vi "Autonomous Independent.vi"() -> ()   [LabVIEW 2019]
doc: "This VI is called when autonomous begins, and will automatically be terminated when autonomous ends. You can carry out timed or sensor driven robot movement independently without needing to return to the caller."
uses:
  <vilib>/Rock Robotics/Network Tables/NT Read String.vi
  Refnums.vi
  <vilib>/Rock Robotics/WPI/ThirdParty/Phoenix-LabVIEW/Motor Controller/Get/CTRE_Phoenix_MotorController_GetQuadratureData.vi
  <vilib>/addons/control/pid/pid.llb/PID (DBL).vi
  <vilib>/Rock Robotics/WPI/RobotDrive/WPI_RobotDriveArcadeDrive_Standard(NoSaturation).vi
  <vilib>/addons/control/pid/NI_PID_pid.lvlib
panel:
  in  "Autonomous Step":T1(array[cluster]) {"Speed" min=0.0 max=1.0 step=0.01}
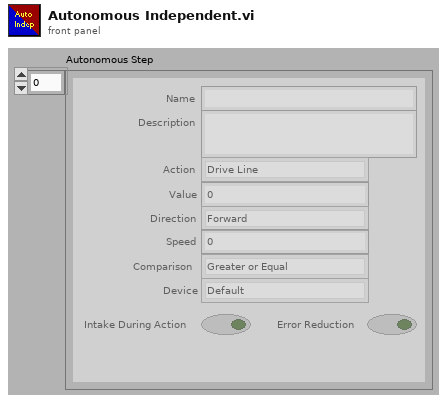
[diagram p1: front panel]
types:
  T1 = cluster{"Name":string, "Description":string, "Action":enum16{"Drive Line", "Drive Turn", "Drive Stop", "Drive Wait", "Shoot", "Motion Profile", ""}, "Value":dbl, "Direction":enum16{"Forward", "Reverse", "Left", "Right"}, "Speed":dbl, "Comparison":enum16{"Greater or Equal", "Less or Equal", "No compare (fixed)"}, "Device":enum16{"Default", "Gyro", "Laser", "Lidar", "Lime Light", "Encoder"}, "Intake During Action":bool, "Error Reduction":bool}[]
  T2 = typedef "WPI_RobotDriveDevRef.ctl" = cluster{"DevStatus":errorcluster, "Motors[]":T3[], "Square Inputs":bool, "Max Output":dbl}
  T3 = typedef "WPI_MotorControlDeviceRef.ctl" = cluster{"DeviceStatus":errorcluster, "Type":T4, "PWM":cluster{"PWM Channel":T5, "DeadBand":T6}, "CAN":cluster{"Device Number":u8, "SetOutput VI Ref":variant, "GetOutput VI Ref":variant, "Enable VI Ref":variant, "Disable VI Ref":variant, "Data":variant}, "Invert":bool, "DIO PWM":cluster{"PWM \"Enable\" Channel":T5, "DIOChannel":T7, "PWM Rate":dbl}}
  T4 = typedef "WPI_MotorControlType.ctl" = enum16{"PWM", "CAN", "DIO PWM"}
  T5 = typedef "FPGA_DIOPWMChannel.ctl" = enum8{"PWM 0", "PWM 1", "PWM 2", "PWM 3", "PWM 4", "PWM 5", "PWM 6", "PWM 7", "PWM 8", "PWM 9", "PWM MXP 0", "PWM MXP 1", "PWM MXP 2", "PWM MXP 3", "PWM MXP 4", "PWM MXP 5", "PWM MXP 6", "PWM MXP 7", "PWM MXP 8", "PWM MXP 9", "Invalid"}
  T6 = typedef "WPI_PWMDeadband.ctl" = cluster{"Name":string, "maxPositivePwm":i32, "minPositivePwm":i32, "centerPwm":i32, "maxNegativePwm":i32, "minNegativePwm":i32, "angularRange":u16}
  T7 = typedef "FPGA_DIOChannel.ctl" = enum8{"DIO 0", "DIO 1", "DIO 2", "DIO 3", "DIO 4", "DIO 5", "DIO 6", "DIO 7", "DIO 8", "DIO 9", "DIO MXP 0", "DIO MXP 1", "DIO MXP 2", "DIO MXP 3", "DIO MXP 4", "DIO MXP 5", "DIO MXP 6", "DIO MXP 7", "DIO MXP 8", "DIO MXP 9", "DIO MXP 10", "DIO MXP 11", "DIO MXP 12", "DIO MXP 13", "DIO MXP 14", "DIO MXP 15", "SPI Port CS1", "SPI Port CS2", "SPI Port CS3", "SPI Port MISO", "SPI Port MOSI", "Invalid"}
  T8 = cluster{"ROBOT_DRIVE":T2, "SHOOTER":T3, "RIGHT_DRIVE":T3, "LEFT_DRIVE":T3, "TURRET":T3, "SHOOTER SLAVE":T3, "INTAKE PIVOT":T3}
  T9 = cluster{"proportional gain (Kc)":dbl, "integral time (Ti, min)":dbl, "derivative time (Td, min)":dbl}
  T10 = enum16{"Drive Line", "Drive Turn", "Drive Stop", "Drive Wait", "Shoot", "Motion Profile", ""}
  T11 = enum16{"Greater or Equal", "Less or Equal", "No compare (fixed)"}
  T12 = enum16{"Default", "Gyro", "Laser", "Lidar", "Lime Light", "Encoder"}
  T13 = cluster{"Yaw":dbl, "Roll":dbl, "Pitch":dbl, "Heading":dbl, "Fused Heading":dbl}
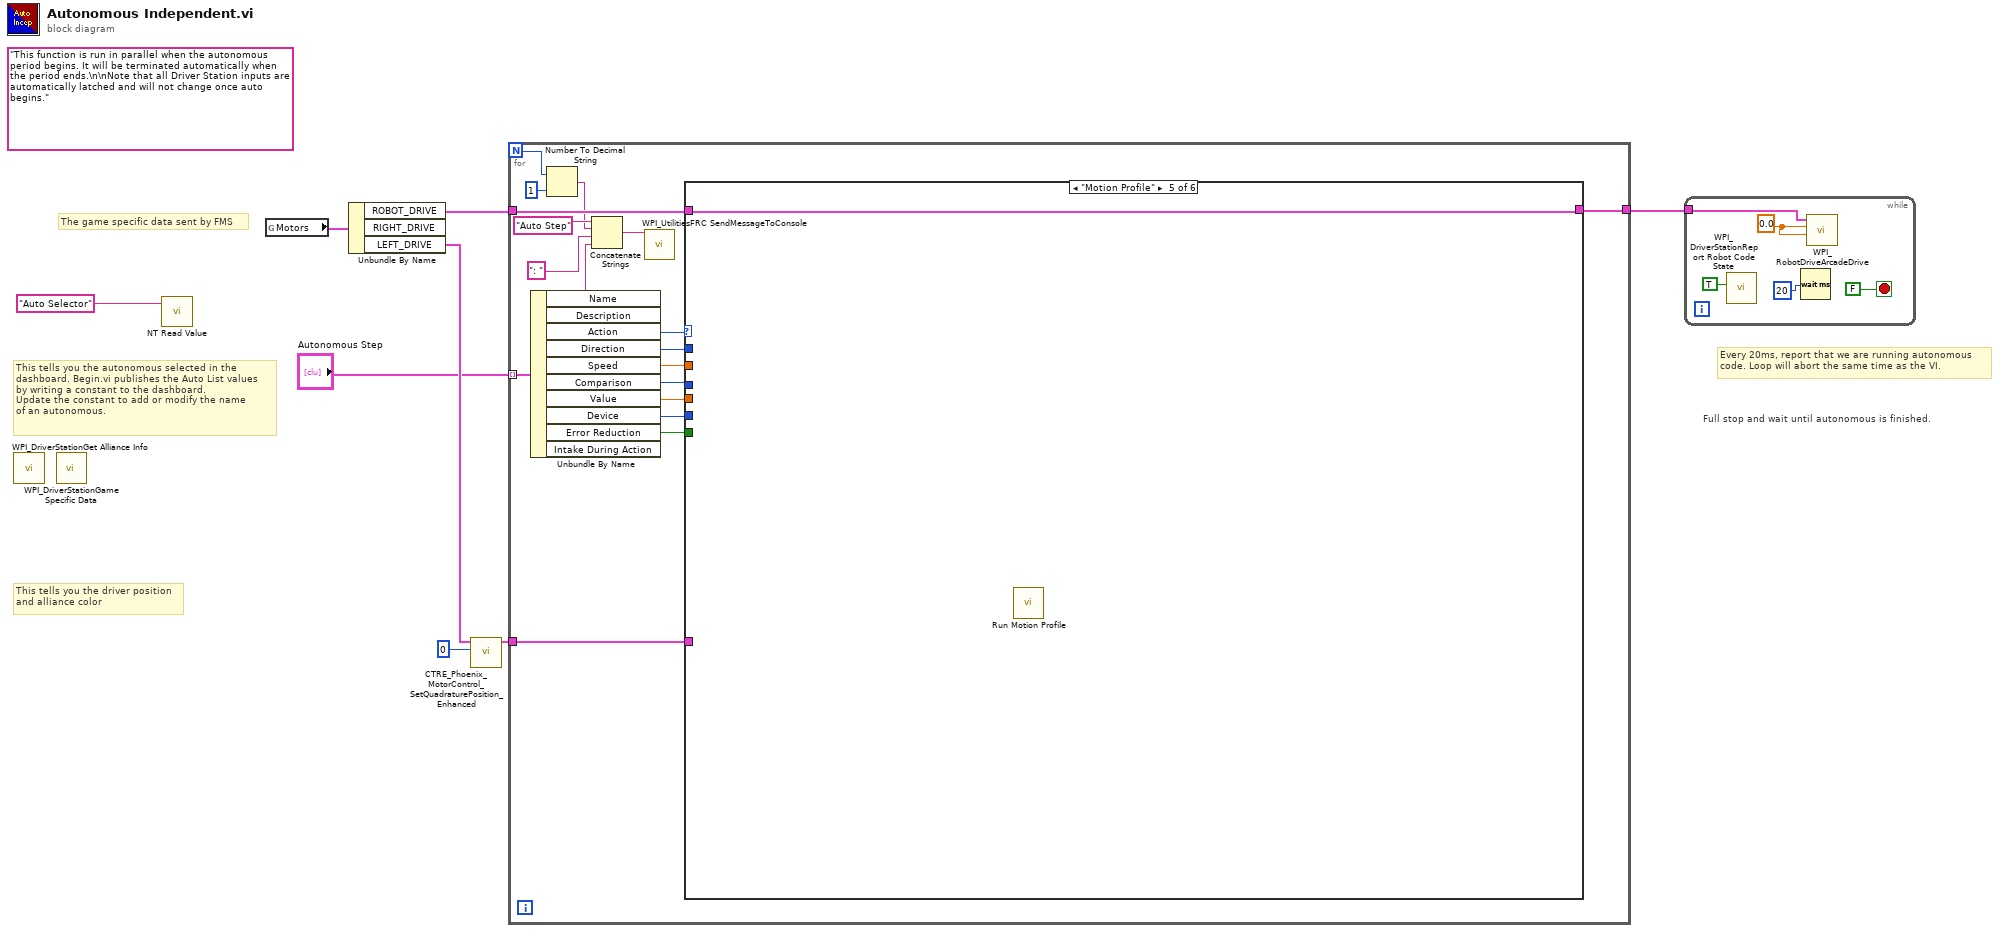
[diagram p0: block diagram]
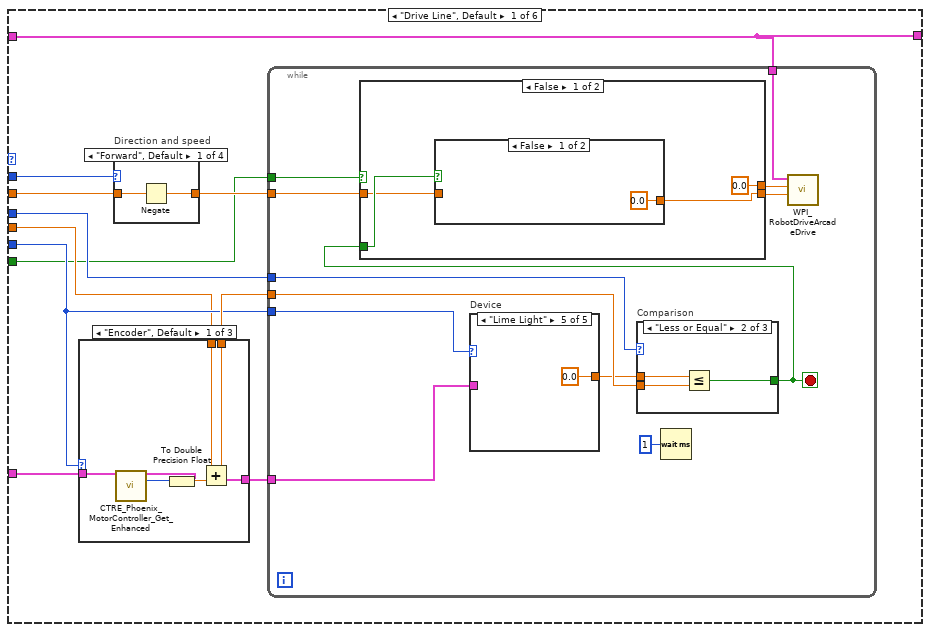
[diagram p2: hidden frame]
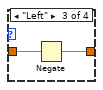
[diagram p6: hidden frame]
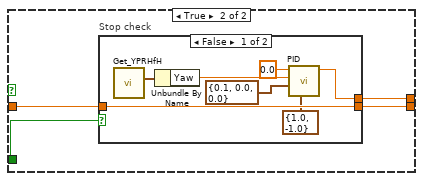
[diagram p9: hidden frame]
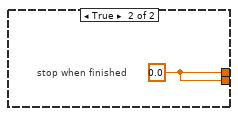
[diagram p10: hidden frame]
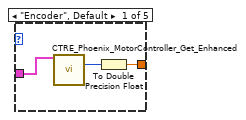
[diagram p11: hidden frame]
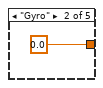
[diagram p12: hidden frame]
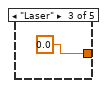
[diagram p13: hidden frame]
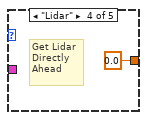
[diagram p14: hidden frame]
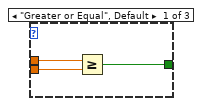
[diagram p15: hidden frame]
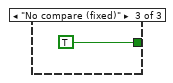
[diagram p16: hidden frame]
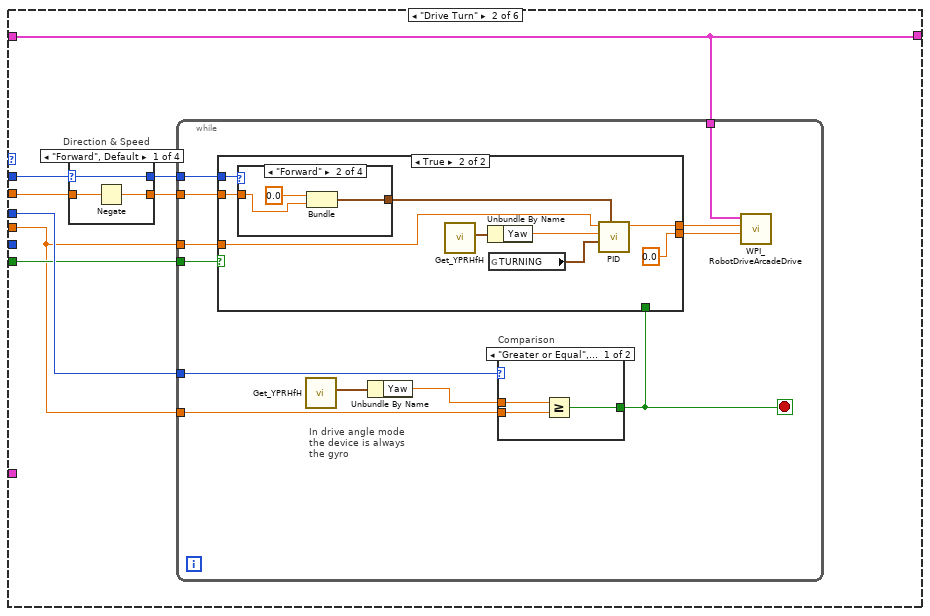
[diagram p17: hidden frame]
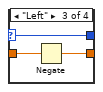
[diagram p19: hidden frame]
diagram:
  (unwired) "This function is run in parallel when the autonomous period begins. It will be terminated automatically when the period ends.\n\nNote that all Driver Station inputs are automatically latched and will not change once auto begins."
  # "Full stop and wait until autonomous is finished."
  # "The game specific data sent by FMS"
  # "This tells you the autonomous selected in the \ndashboard. Begin.vi publishes the Auto List values\nby writing a constant to the dashboard.\nUpdate the constant to add or modify the name\nof an autonomous."
  # "Every 20ms, report that we are running autonomous\ncode. Loop will abort the same time as the VI."
  # "This tells you the driver position\nand alliance color"
  n1 = call <vilib>:"WPI_DriverStationGet Alliance Info.vi"() -> ()  [unwired: 12 out]
  n2 = call <vilib>:"WPI_DriverStationGame Specific Data.vi"() -> ()  [unwired: 11 in, 1 out]
  n3 = call-poly <vilib>:"NT Read Value.vi"("Name"="Auto Selector") -> ()  [unwired: 9 in, 2 out]
  n4 = global read "Refnums.vi" "Motors"() -> (w7:T8)
  n5 = Unbundle By Name(w7) -> ("ROBOT_DRIVE"=w4:T2, "LEFT_DRIVE"=w2:T3)  [unwired: 1 out]
  n6 = call <vilib>:"CTRE_Phoenix_MotorControl_SetQuadraturePosition_Enhanced.vi"("New Position"=0, "PhoenixMotorControlDevRef"=w2) -> ("PhoenixMotorControlDevRef"=w5:T3)  [unwired: 8 in, 1 out]
  n7 = for {
    N -> [w11]
    tunnel: "Autonomous Step" -> [w26] mode=indexing
    tunnel: w5 -> [w18]
    tunnel: w4 -> [w17]
    tunnel: [w16] -> w3
    n8 = Unbundle By Name(w26) -> ("Name"=w14:string, "Action"=w25:T10, "Direction"=w24:enum16{"Forward", "Reverse", "Left", "Right"}, "Speed"=w23:dbl, "Comparison"=w19:T11, "Value"=w20:dbl, "Device"=w22:T12, "Error Reduction"=w21:bool)  [unwired: 2 out]
    n9 = Number To Decimal String(number=w11, width (-)=i16 1) -> (decimal integer string=w9:string)
    n10 = Concatenate Strings("Auto Step" ("string"), w9, ": " ("string"), w14) -> (w15:string)
    n11 = call <vilib>:"WPI_UtilitiesFRC SendMessageToConsole.vi"("Message"=w15) -> ()  [unwired: 14 in, 1 out]
    n12 = case shown="\"Motion Profile\"" w25 {
      tunnel: w24 -> [w32 w102 _ _ _ _]
      tunnel: w23 -> [w33 w104 _ _ _ _]
      tunnel: w22 -> [w34 _ _ _ _ _]
      tunnel: w21 -> [w27 w100 _ _ _ _]
      tunnel: w20 -> [w31 w98 _ w164 _ _]
      tunnel: w19 -> [w30 w103 _ _ _ _]
      tunnel: w18 -> [w29 _ _ _ _ _]
      tunnel: w17 -> [w28 w101 w162 w165 w166 w167]
      tunnel: [w28 w101 w162 w165 w166 w167] -> w16
      frame "Drive Line", Default {
        n13 = case shown="\"Encoder\", Default" w34 {
          tunnel: w29 -> [w43 w44 w46]
          tunnel: w31 -> [w40 w45 w47]
          tunnel: [w39 w45 w47] -> w36
          tunnel: [w38 w44 w46] -> w35
          frame "Encoder", Default {
            n14 = call-poly <vilib>:"CTRE_Phoenix_MotorController_Get_Enhanced.vi"("PhoenixMotorControlDevRef"=w43) -> ("PhoenixMotorControlDevRef"=w38:T3, "Quadrature Position"=w41:i32)  [unwired: 11 in, 2 out]
            n15 = To Double Precision Float(number=w41) -> (double precision float=w42:dbl)
            n16 = Add(x=w40, y=w42) -> (x+y=w39:dbl)
          }
          frame "Gyro" {
          }
          frame "Laser" {
          }
        }
        n17 = case "Direction and speed" shown="\"Forward\", Default" w32 {
          tunnel: w33 -> [w48 w50 w51 w53]
          tunnel: [w49 w50 w52 w53] -> w37
          frame "Forward", Default {
            n18 = Negate(x=w48) -> (-x=w49:dbl)
          }
          frame "Reverse" {
          }
          frame "Left" {
            n19 = Negate(x=w51) -> (-x=w52:dbl)
          }
          frame "Right" {
          }
        }
        n20 = while {
          tunnel: w30 -> [w60]
          tunnel: w36 -> [w65]
          tunnel: w37 -> [w64]
          tunnel: w34 -> [w59]
          tunnel: w28 -> [w61]
          tunnel: w35 -> [w57]
          tunnel: w27 -> [w54]
          stop <- w55 stop-if-true
          n21 = case "Device" shown="\"Lime Light\"" w59 {
            tunnel: [w85 0.0 0.0 0.0 0.0] -> w58
            tunnel: w57 -> [w86 _ _ _ _]
            frame "Encoder", Default {
              n22 = call-poly <vilib>:"CTRE_Phoenix_MotorController_Get_Enhanced.vi"("PhoenixMotorControlDevRef"=w86) -> ("Quadrature Position"=w84:i32)  [unwired: 11 in, 3 out]
              n23 = To Double Precision Float(number=w84) -> (double precision float=w85:dbl)
            }
            frame "Gyro" {
            }
            frame "Laser" {
            }
            frame "Lidar" {
              # "Get Lidar \nDirectly \nAhead"
            }
            frame "Lime Light" {
            }
          }
          n24 = case "Comparison" shown="\"Less or Equal\"" w60 {
            tunnel: [w93 w96 TRUE] -> w55
            tunnel: w65 -> [w92 w95 _]
            tunnel: w58 -> [w91 w94 _]
            frame "Greater or Equal", Default {
              n25 = Greater Or Equal?(x=w91, y=w92) -> (x >= y?=w93:bool)
            }
            frame "Less or Equal" {
              n26 = Less Or Equal?(x=w94, y=w95) -> (x <= y?=w96:bool)
            }
            frame "No compare (fixed)" {
            }
          }
          n27 = case shown="False" w54 {
            tunnel: w64 -> [w67 w75]
            tunnel: [0.0 ("X axis value") w74] -> w63
            tunnel: [w66 w73] -> w62
            tunnel: w55 -> [w68 w72]
            frame False {
              n28 = case shown="False" w68 {
                tunnel: w67 -> [_ w71]
                tunnel: [0.0 ("Speed") w71] -> w66
                frame False {
                }
                frame True {
                }
              }
            }
            frame True {
              n29 = case "Stop check" shown="False" w72 {
                tunnel: w75 -> [w82 _]
                tunnel: [w81 w83] -> w74
                tunnel: [w82 w83] -> w73
                frame False {
                  n30 = call <vilib>:"Get_YPRHfH.vi"() -> ("YRPHfH"=w77:T13)  [unwired: 11 in]
                  n31 = Unbundle By Name(w77) -> ("Yaw"=w76:dbl)
                  n32 = call-poly <vilib>:"PID.vi"("output range"=cluster{"output high":dbl, "output low":dbl} {"output high"=1.0, "output low"=-1.0}, "PID gains"=T9 {"proportional gain (Kc)"=0.1, "integral time (Ti, min)"=0.0, "derivative time (Td, min)"=0.0}, "process variable"=w76, "setpoint"=0.0) -> ("output"=w81:dbl)  [unwired: 6 in, 1 out]
                }
                frame True {
                  w83 = 0.0 ("X axis value")
                  # "stop when finished"
                }
              }
            }
          }
          n33 = Wait (ms)(milliseconds to wait=u32 1) -> ()  [unwired: 1 out]
          n34 = call-poly <vilib>:"WPI_RobotDriveArcadeDrive.vi"("Y axis value"=w62, "X axis value"=w63, "RobotDriveDevRef"=w61) -> ()  [unwired: 1 in, 8 out]
        }
      }
      frame "Drive Turn" {
        n35 = case "Direction & Speed" shown="\"Forward\", Default" w102 {
          selector: w102 -> [w106 w109 w111 w114]
          tunnel: w104 -> [w107 w110 w112 w115]
          tunnel: [w108 w110 w113 w115] -> w105
          tunnel: [w106 w109 w111 w114] -> w99
          frame "Forward", Default {
            n36 = Negate(x=w107) -> (-x=w108:dbl)
          }
          frame "Reverse" {
          }
          frame "Left" {
            n37 = Negate(x=w112) -> (-x=w113:dbl)
          }
          frame "Right" {
          }
        }
        n38 = while {
          tunnel: w103 -> [w120]
          tunnel: w98 -> [w119]
          tunnel: w105 -> [w127]
          tunnel: w101 -> [w124]
          tunnel: w100 -> [w123]
          tunnel: w99 -> [w118]
          tunnel: w98 -> [w117]
          stop <- w116 stop-if-true
          # "In drive angle mode\nthe device is always\nthe gyro"
          n39 = call <vilib>:"Get_YPRHfH.vi"() -> ("YRPHfH"=w121:T13)  [unwired: 11 in]
          n40 = Unbundle By Name(w121) -> ("Yaw"=w122:dbl)
          n41 = case "Comparison" shown="\"Greater or Equal\", Default" w120 {
            tunnel: [w130 w133] -> w116
            tunnel: w122 -> [w129 w132]
            tunnel: w119 -> [w128 w131]
            frame "Greater or Equal", Default {
              n42 = Greater Or Equal?(x=w129, y=w128) -> (x >= y?=w130:bool)
            }
            frame "Less or Equal" {
              n43 = Less Or Equal?(x=w132, y=w131) -> (x <= y?=w133:bool)
            }
          }
          n44 = case shown="True" w123 {
            tunnel: w127 -> [w137 w149]
            tunnel: [w136 w144] -> w126
            tunnel: [w135 0.0 ("X axis value")] -> w125
            tunnel: w118 -> [_ w142]
            tunnel: w117 -> [_ w141]
            tunnel: w116 -> [w134 _]
            frame False {
              n45 = case shown="False" w134 {
                tunnel: w137 -> [w139 _]
                tunnel: [w139 w140] -> w136
                tunnel: [0.0 ("X axis value") w140] -> w135
                frame False {
                }
                frame True {
                  w140 = 0.0 ("X axis value")
                }
              }
            }
            frame True {
              n46 = case shown="\"Forward\"" w142 {
                tunnel: w149 -> [w150 w155 w157 w161]
                tunnel: [w152 w153 w156 w159] -> w148
                frame "Reverse" {
                  n47 = Bundle("Speed"=w150, 0.0) -> (w152:cluster{"Speed":dbl, dbl})  [unwired: 1 in]
                }
                frame "Forward" {
                  n48 = Bundle(0.0, "Speed"=w155) -> (w153:cluster{dbl, "Speed":dbl})  [unwired: 1 in]
                }
                frame "Right", Default {
                  n49 = Bundle("Speed"=w157, 0.0) -> (w156:cluster{"Speed":dbl, dbl})  [unwired: 1 in]
                }
                frame "Left" {
                  n50 = Bundle(0.0, "Speed"=w161) -> (w159:cluster{dbl, "Speed":dbl})  [unwired: 1 in]
                }
              }
              n51 = call <vilib>:"Get_YPRHfH.vi"() -> ("YRPHfH"=w147:T13)  [unwired: 11 in]
              n52 = Unbundle By Name(w147) -> ("Yaw"=w146:dbl)
              n53 = global read "PID.vi" "TURNING"() -> (w145:cluster{"P":dbl, "I":dbl, "D":dbl})
              n54 = call-poly <vilib>:"PID.vi"("output range"=w148, "PID gains"=w145, "process variable"=w146, "setpoint"=w141) -> ("output"=w144:dbl)  [unwired: 6 in, 1 out]
            }
          }
          n55 = call-poly <vilib>:"WPI_RobotDriveArcadeDrive.vi"("Y axis value"=w125, "X axis value"=w126, "RobotDriveDevRef"=w124) -> ()  [unwired: 1 in, 8 out]
        }
      }
      frame "Drive Stop" {
        w163 = 0.0 ("X axis value")
        # "Stop all drive motion"
        n56 = call-poly <vilib>:"WPI_RobotDriveArcadeDrive.vi"("Y axis value"=w163, "X axis value"=w163, "RobotDriveDevRef"=w162) -> ()  [unwired: 1 in, 8 out]
      }
      frame "Drive Wait" {
        n57 = call <vilib>:"WPI_RobotDriveDelayAndUpdateSafety.vi"("Delay (s)"=w164, "RobotDriveDevRef"=w165) -> ()  [unwired: 8 in, 2 out]
      }
      frame "Motion Profile" {
        n58 = call "Run Motion Profile.vi"() -> ()  [unwired: 12 in]
      }
      frame "Shoot" {
      }
    }
  }
  n59 = while {
    tunnel: w3 -> [w169]
    stop <- FALSE stop-if-true
    w168 = 0.0 ("X axis value")
    n60 = call <vilib>:"WPI_DriverStationReport Robot Code State.vi"("Autonomous"=TRUE) -> ()  [unwired: 10 in, 1 out]
    n61 = Wait (ms)(milliseconds to wait=u32 20) -> ()  [unwired: 1 out]
    n62 = call-poly <vilib>:"WPI_RobotDriveArcadeDrive.vi"("Y axis value"=w168, "X axis value"=w168, "RobotDriveDevRef"=w169) -> ()  [unwired: 6 in, 3 out]
  }
